vi "Anritsu VNA Read Power.vi"(6 "Channel":i8=1 min=1 max=99 step=1, 7 "Anritsu VNA":T1, 8 "error in (no error)":errorcluster, 11 "VISA Resource Name":refnum<visa-resource-name>) -> (0 "error out":errorcluster, 2 "Source Power, dBm":dbl, 3 "dup VISA Resource Name":refnum<visa-resource-name>)   [LabVIEW 2011]
doc: "This vi sets the power range. Only works on the HP 8753D."
uses:
  TypeDefs/Anritsu VNA Instrument Info.ctl
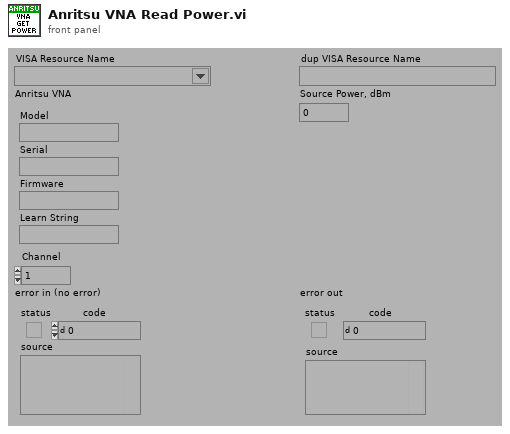
[diagram p1: front panel]
types:
  T1 = typedef "Anritsu VNA Instrument Info.ctl" = cluster{"Model":string, "Serial":string, "Firmware":string, "Learn String":string}
  T2 = typedef "Anritsu VNA Model.ctl" = enum16{"Not Supported", "37XXXX", "MS20XXX", "MS462XX", "MS464XX"}
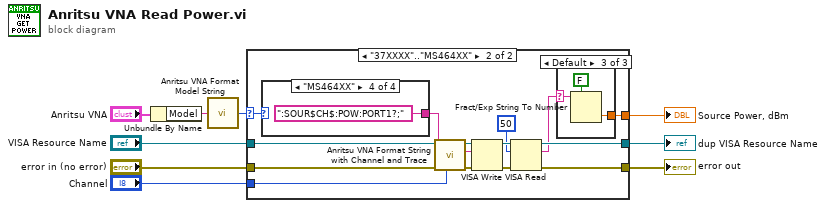
[diagram p0: block diagram]
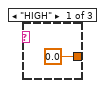
[diagram p3: hidden frame]
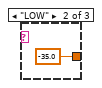
[diagram p4: hidden frame]
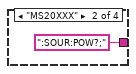
[diagram p6: hidden frame]
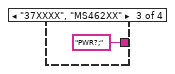
[diagram p7: hidden frame]
diagram:
  n1 = Unbundle By Name("Anritsu VNA") -> ("Model"=w3:string)
  n2 = call "Anritsu VNA Format Model String.vi"("Model"=w3) -> ("Model"=w2:T2)
  n3 = case shown="\"37XXXX\"..\"MS464XX\"" w2 {
    selector: w2 -> [_ w15]
    tunnel: "VISA Resource Name" -> [w11 w24]
    tunnel: "error in (no error)" -> [w10 w23]
    tunnel: [w11 w21] -> w7
    tunnel: [w10 w19] -> w6
    tunnel: [_ w16] -> w4
    tunnel: "Channel" -> [_ w12]
    frame "Not Supported" {
    }
    frame "37XXXX".."MS464XX" {
      n4 = case shown="\"MS464XX\"" w15 {
        tunnel: [_ ":SOUR:POW?;" "PWR?;" ":SOUR$CH$:POW:PORT1?;"] -> w13
        frame "Not Supported" {
        }
        frame "MS20XXX" {
        }
        frame "37XXXX", "MS462XX" {
        }
        frame "MS464XX" {
        }
      }
      n5 = call "Anritsu VNA Format String with Channel and Trace.vi"("Channel"=w12, "String"=w13) -> ("String Out"=w14:string)  [unwired: 1 in, 6 out]
      n6 = VISA Write(VISA resource name=w24, write buffer=w14, error in (no error)=w23) -> (VISA resource name out=w22:refnum<visa-resource-name>, error out=w20:errorcluster)  [unwired: 1 out]
      n7 = VISA Read(VISA resource name=w22, byte count=u32 50, error in (no error)=w20) -> (VISA resource name out=w21:refnum<visa-resource-name>, read buffer=w17:string, error out=w19:errorcluster)  [unwired: 1 out]
      n8 = case shown="Default" w17 {
        selector: w17 -> [_ _ w28]
        tunnel: [0.0 ("Source Power, dBm") -35.0 ("Source Power, dBm") w27] -> w16
        frame "HIGH" {
        }
        frame "LOW" {
        }
        frame Default {
          n9 = Fract/Exp String To Number(use system decimal point (T)=FALSE, string=w28) -> (number=w27:dbl)  [unwired: 3 out]
        }
      }
    }
  }
  "dup VISA Resource Name" <- w7
  "error out" <- w6
  "Source Power, dBm" <- w4
